vi "image taking.vi"() -> ()   [LabVIEW 2021]
uses:
  <vilib>/userdefined/High Color/IMAQdx.ctl
  <vilib>/vision/driver/NI_Vision_Acquisition_Software.lvlib
panel:
  out "error out 4":errorcluster
  out "error out 3":errorcluster
  out "error out 2":errorcluster
  in  "take image":bool
  in  "stop":bool
  out "Image":T1(plugin-control)
  out "error out":errorcluster
  in  "Session In":T2
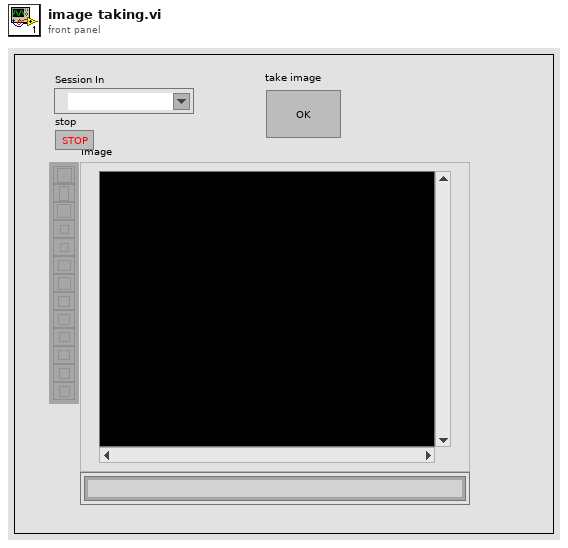
[diagram p1: front panel]
types:
  T1 = typedef "IMAQ Image.ctl" = refnum<image>
  T2 = typedef "IMAQdx.ctl" = refnum<k21>
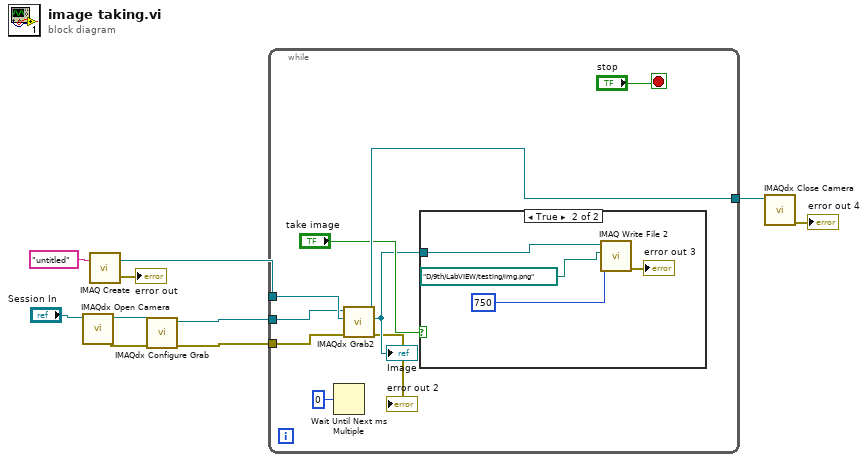
[diagram p0: block diagram]
diagram:
  n1 = call <vilib>:"IMAQdx Open Camera.vi"("Session In"="Session In") -> ("error out"=w6:errorcluster, "Session Out"=w5:T2)  [unwired: 9 in]
  n2 = call "IMAQ Create"("Image Name"="untitled") -> ("New Image"=w8:T1, "error out"=→"error out":errorcluster)  [unwired: 4 in]
  n3 = call <vilib>:"IMAQdx Configure Grab.vi"("error in"=w6, "Session In"=w5) -> ("error out"=w4:errorcluster, "Session Out"=w3:T2)  [unwired: 8 in]
  n4 = while {
    tunnel: w8 -> [w18]
    tunnel: w4 -> [w17]
    tunnel: w3 -> [w16]
    tunnel: [w15] -> w2
    stop <- "stop" stop-if-true
    n5 = Wait Until Next ms Multiple(millisecond multiple=u32 0) -> ()  [unwired: 1 out]
    n6 = call <vilib>:"IMAQdx Grab2.vi"("error in"=w17, "Image In"=w18, "Session In"=w16) -> ("error out"=→"error out 2":errorcluster, "Image Out"=w12:T1, "Session Out"=w15:T2)  [unwired: 5 in, 1 out]
    "Image" <- w12
    n7 = case shown="True" "take image" {
      tunnel: w12 -> [_ w23]
      frame False {
      }
      frame True {
        n8 = call-poly "IMAQ Write File 2"("Image Quality"=u32 750, "File Path"=path "D:/9th/LabVIEW/testing/img.png", "Image"=w23) -> ("error out"=→"error out 3":errorcluster)  [unwired: 7 in, 1 out]
      }
    }
  }
  n9 = call <vilib>:"IMAQdx Close Camera.vi"("Session In"=w2) -> ("error out"=→"error out 4":errorcluster)  [unwired: 10 in]
